vi "test_SetName.vi"   [LabVIEW 2013]
uses:
  source/TypeDescriptor/TypeDescriptor_SetName.vi
  source/Variant/OpenVariant.lvlib
types:
  T1 = typedef "Semaphore RefNum" = refnum<k1>
  T2 = cluster{"This is the boolean item's name":bool, "BBB":i32, "CCCC":string, "Data":dbl}
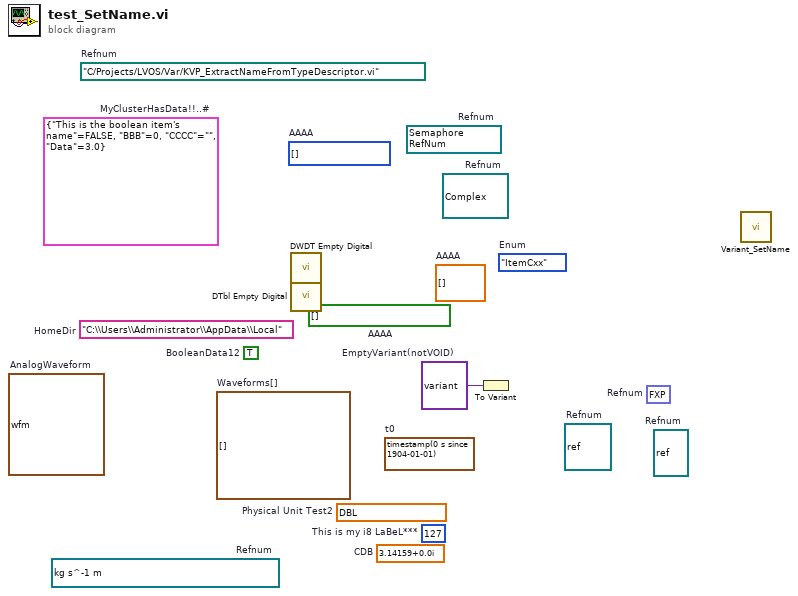
[diagram p0: block diagram]
diagram:
  (unwired) fxp<+,7,7> 127.0  # Refnum
  (unwired) refnum<class> refnum  # Refnum
  w1 = variant  # EmptyVariant(notVOID)
  (unwired) timestamp(0 s since 1904-01-01)  # t0
  (unwired) waveform(dbl)[] []  # Waveforms[]
  (unwired) bool[] []  # AAAA
  (unwired) refnum<notifier> refnum items=["Item1", "Item2", "Item3A"]  # Refnum
  (unwired) T1 refnum items=["semaphore"]  # Refnum
  (unwired) refnum<queue> refnum  # Refnum
  (unwired) refnum<vi> refnum  # Refnum
  (unwired) waveform(dbl) {"t0"=timestamp(0 s since 1904-01-01), "dt"=1.0, "Y"=[]}  # AnalogWaveform
  (unwired) dbl[][] []  # AAAA
  (unwired) enum8{"Item1", "Item2", "Item3A"}[] [] items=["Item1", "Item2", "Item3A"]  # AAAA
  (unwired) cxt[unit] 3.141590118408203+0.0i  # Physical Unit Test2
  (unwired) path "C:/Projects/LVOS/Var/KVP_ExtractNameFromTypeDescriptor.vi"  # Refnum
  (unwired) T2 {"This is the boolean item's name"=FALSE, "BBB"=0, "CCCC"="", "Data"=3.0}  # MyClusterHasData!!..#
  (unwired) enum8{"A", "B2\ntest", "ItemCxx"}."ItemCxx"  # Enum
  (unwired) "C:\\Users\\Administrator\\AppData\\Local"  # HomeDir
  (unwired) TRUE  # BooleanData12
  (unwired) i8 127  # This is my i8 LaBeL***
  (unwired) cdb 3.14159+0.0i  # CDB
  n1 = call <vilib>:"DWDT Empty Digital.vi"() -> ()  [unwired: 5 in, 1 out]
  n2 = call <vilib>:"DTbl Empty Digital.vi"() -> ()  [unwired: 5 in, 1 out]
  n3 = To Variant(anything=w1) -> ()  [unwired: 1 out]
  n4 = call "Variant_SetName.vi"() -> ()  [unwired: 11 in, 1 out]
